vi "UiGascounter.vi"() -> ()   [LabVIEW 2011]
uses:
  Output - Cluster b2g1.ctl
  <vilib>/Platform/TimedLoop/XDataNode/timing_clust.ctl
  <vilib>/Platform/TimedLoop/XDataNode/nitl_modes.ctl
  <vilib>/Platform/TimedLoop/XDataNode/wakeup.ctl
  <vilib>/Platform/TimedLoop/XDataNode/XDataNode.xnode
  <vilib>/Platform/TimedLoop/XDataNode/XDNodeRunTimeDep.lvlib
panel:
  out "Volumen [l]":dbl format="%.2f"
  in  "stop":bool
  out "TS-6 [°C]":dbl format="%.2g"
  out "Impulse":u64
  out "DS-3 [bar]":dbl format="%.5g"
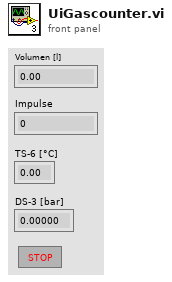
[diagram p1: front panel]
types:
  T1 = typedef "Output - Cluster b2g1.ctl" = cluster{"DFS-1 [dl]":u64, "FS-3 [l]":dbl, "DFS-1 [l/min]":dbl, "DS-1 [bar]":dbl, "V-10 ZU":bool, "V-14 ZU":bool, "FS-1 [l]":dbl, "FS-2 [l]":dbl, "TS-4 [°C]":dbl, "HS-1":bool, "V-13 [%]":u8, "V-15 [%]":u8, "P-4 [%]":u8, "P-5 [%]":u8, "Dosierung":bool, "MR Max Füllstand":bool, "MR Min Füllstand":bool, "Dosiermenge [l]":sgl, "V-14 AUF":bool, "V-10 AUF":bool, "T-1 Max Füllstand":bool, "T-1 Min Füllstand":bool, "T-2 Max Füllstand":bool, "T-2 Min Füllstand":bool, "pHS-1 [pH]":dbl, "P-4 RUN":bool, "P-5 RUN ":bool, "V-33 AUF":bool, "V-33 ZU":bool, "V-34 AUF":bool, "V-34 ZU":bool, "P-4 ERR":bool, "P-5 ERR":bool, "TS-5 [°C]":dbl, "GZ-1 [dl]":u64, "TS-6 [°C]":dbl, "DS-3 [bar]":dbl, "P-9 RUN":bool}
  T2 = typedef "XDNodeRunTimeDep.lvlib/timing_clust.ctl" = cluster{"Expected End [f-1]":u64, "Actual End [f-1]":u64, "Finished Late? [f-1]":bool, "Expected End [i-1]":u64, "Actual End [i-1]":u64, "Finished Late? [i-1]":bool, "Expected Start [i]":u64, "Actual Start [i]":u64, "Expected Start [f]":u64, "Actual Start [f]":u64, "Source Name":string, "Structure Name":string, "Period":i64, "Deadline":i64, "Offset":i64, "Start":i64, "Priority":i32, "Timeout":i32, "Mode":T3, "Wakeup Reason":T4, "Error":errorcluster, "Source Type":string, "Secondary Source Type":string, "Global End Time":u64, "Global Start Time":u64, "Frame Duration":u64, "Iteration Duration":u64, "Assigned CPU":i32, "I/O Scan Engine Mode":u32}
  T3 = typedef "XDNodeRunTimeDep.lvlib/nitl_modes.ctl" = enum32{"No Change", "Process missed periods, maintain original phase", "Discard missed periods, maintain original phase", "Process missed periods, ignore original phase", "Discard missed periods, ignore original phase"}
  T4 = typedef "XDNodeRunTimeDep.lvlib/wakeup.ctl" = enum32{"Normal", "Aborted", "Asynchronous wakeup", "Timing source error", "Timed loop error", "Timeout"}
  T5 = enum32{"invalid app kind", "Development System", "Run Time System", "Student Edition", "Embedded LabVIEW", "Evaluation", "Custom"}
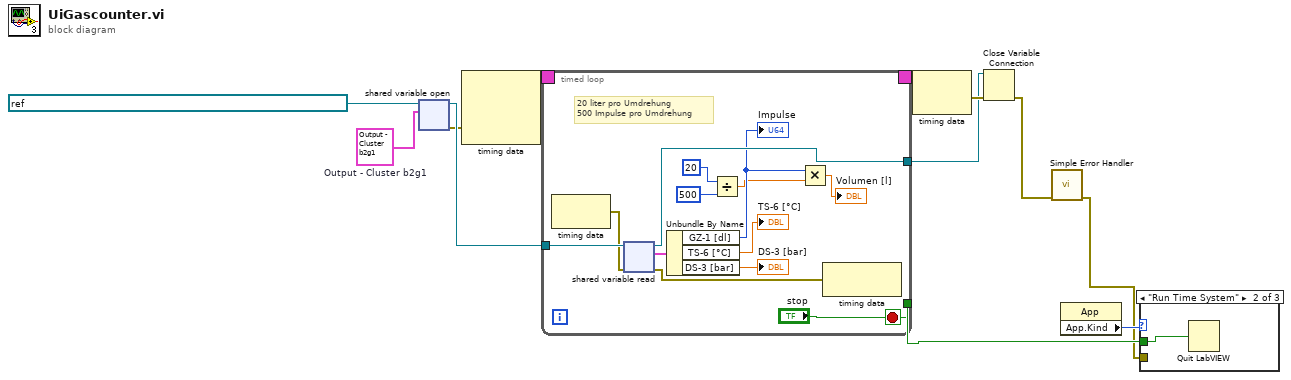
[diagram p0: block diagram]
diagram:
  w10 = T1 {"DFS-1 [dl]"=0, "FS-3 [l]"=0.0, "DFS-1 [l/min]"=0.0, "DS-1 [bar]"=0.0, "V-10 ZU"=FALSE, "V-14 ZU"=FALSE, "FS-1 [l]"=0.0, "FS-2 [l]"=0.0, "TS-4 [°C]"=0.0, "HS-1"=FALSE, "V-13 [%]"=0, "V-15 [%]"=0, "P-4 [%]"=0, "P-5 [%]"=0, "Dosierung"=FALSE, "MR Max Füllstand"=FALSE, "MR Min Füllstand"=FALSE, "Dosiermenge [l]"=0.0, "V-14 AUF"=FALSE, "V-10 AUF"=FALSE, "T-1 Max Füllstand"=FALSE, "T-1 Min Füllstand"=FALSE, "T-2 Max Füllstand"=FALSE, "T-2 Min Füllstand"=FALSE, "pHS-1 [pH]"=0.0, "P-4 RUN"=FALSE, "P-5 RUN "=FALSE, "V-33 AUF"=FALSE, "V-33 ZU"=FALSE, "V-34 AUF"=FALSE, "V-34 ZU"=FALSE, "P-4 ERR"=FALSE, "P-5 ERR"=FALSE, "TS-5 [°C]"=0.0, "GZ-1 [dl]"=0, "TS-6 [°C]"=0.0, "DS-3 [bar]"=0.0, "P-9 RUN"=FALSE}  # Output - Cluster b2g1
  n1 = shared-variable-open(refnum<k21> "ni.var.psp://10.27.40.24/variables - b2g1/data - network - b2g1" ("shared variable refnum in"), w10) -> (w11:refnum<k21>, w7:errorcluster)  [unwired: 2 in]
  n2 = node-c288(w7) -> (w9:T2)  [unwired: 2 in]
  n3 = timed-loop {
    timing: w9 -> [_]
    timing-out: [_] -> w8
    tunnel: w11 -> [w25]
    tunnel: [w21] -> w5
    tunnel: ["stop"] -> w3
    stop <- "stop" stop-if-true
    # "20 liter pro Umdrehung\n500 Impulse pro Umdrehung"
    n4 = node-c288() -> (w23:errorcluster)  [unwired: 1 in]
    n5 = shared-variable-read(w25, w23) -> (w21:refnum<k21>, w22:errorcluster, w24:T1)  [unwired: 1 out]
    n6 = Unbundle By Name(w24) -> ("GZ-1 [dl]"=w18:u64, "TS-6 [°C]"=→"TS-6 [°C]":dbl, "DS-3 [bar]"=→"DS-3 [bar]":dbl)
    "Impulse" <- w18
    n7 = Divide(x=20, y=500) -> (x/y=w15:dbl)
    n8 = Multiply(x=w18, y=w15) -> (x*y=→"Volumen [l]":dbl)
    n9 = node-c288(w22) -> ()  [unwired: 1 out]
  }
  n10 = node-c288(w8) -> (w6:errorcluster)
  n11 = Close Variable Connection(8:w6, 11:w5) -> (0:w2:errorcluster)
  n12 = call <vilib>:"Simple Error Handler.vi"("error in (no error)"=w2) -> ("error out"=w1:errorcluster)  [unwired: 4 in, 4 out]
  n13 = property class="App"() -> ("App.Kind"=w4:T5)  [unwired: 2 in, 2 out]
  n14 = case shown="\"Run Time System\"" w4 {
    tunnel: w3 -> [_ w31 _]
    tunnel: w1 -> [_ _ _]
    frame "invalid app kind", Default {
    }
    frame "Run Time System" {
      n15 = Quit LabVIEW(quit? (T)=w31) -> ()
    }
    frame "Development System" {
    }
  }
